vi "QAM Single Carrier.vi"(4 "Symbol Rate":i32=1, 5 "Samples/Symbol":i32, 6 "DataLen":i32, 7 "QAM Comparison":enum16{"MT Modulate", "Homebrew"}(ring), 8 "QAM Complexity":T1(ring)) -> (0 "sampling info":cluster{"Fs":dbl, "#s":dbl}={"Fs"=1000.0, "#s"=1000.0} {"Fs" format="%.2p"}, 1 "Waveform Graph":cluster{"t0":dbl, "dt":dbl, "Y":dbl[]}(graph), 2 "Waveform":waveform(cdb), 3 "Constellation Graph":T2(graph))   [LabVIEW 2018]
uses:
  <vilib>/addons/Modulation/Analog/support/mod_Set Error Source.vi
  <vilib>/Utility/file.llb/Read Delimited Spreadsheet (DBL).vi
  <vilib>/addons/Modulation/Digital/Support/Common/Validators/mod_Generate Filter Coefficients Validate.vi
  <vilib>/addons/Modulation/Digital/General/subVIs/mod_Generate Filter Coefficients.vi
  <vilib>/addons/Modulation/niDMT.lvlib
panel:
  out "size(s)":i32
  out "Array - Numeric":cdb[](array[numeric])
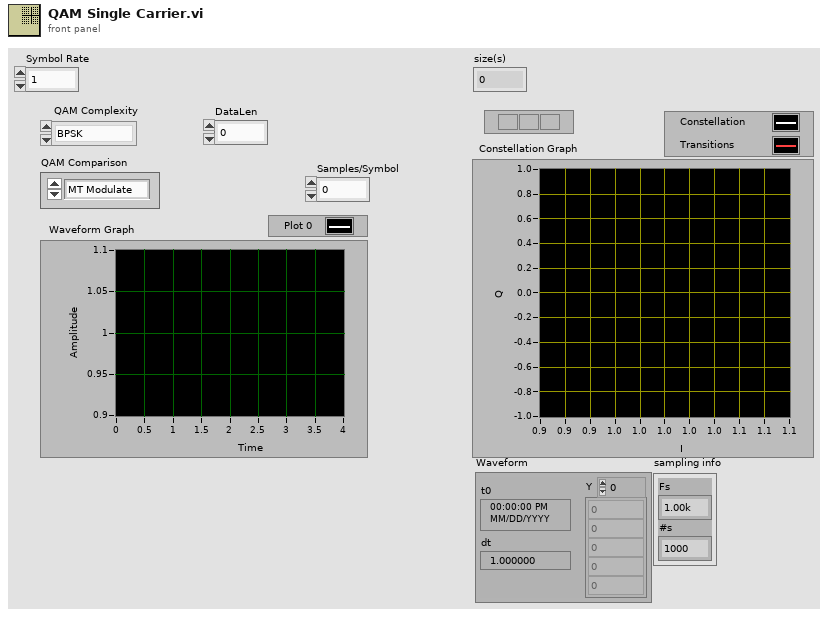
[diagram p1: front panel]
types:
  T1 = enum16{"BPSK", "QPSK", "16-QAM", "64-QAM", "256-QAM"}
  T2 = cluster{"Decimated Array":dbl[], "Decimated Array":dbl[]}[]
  T3 = cluster{"Samples/Symbol":i32, "Array - Numeric":cdb[]}
  T4 = enum16{"FSK", "PSK", "QAM", "MSK", "PAM", "ASK", "CPM"}
  T5 = typedef "niAMT.lvlib/Complex Data Waveform.ctl" = cluster{"t0":dbl, "dt":dbl, "Y":cdb[]}
  T6 = cluster{"constellation":dbl[], "oversampled data":dbl[]}[]
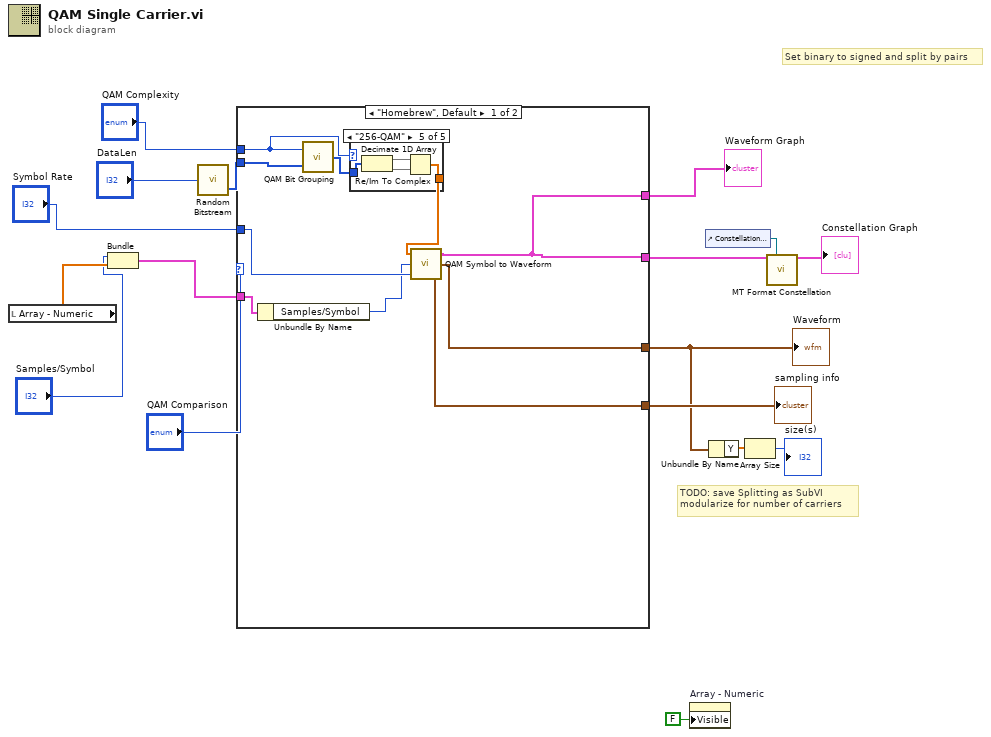
[diagram p0: block diagram]
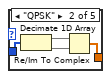
[diagram p3: hidden frame]
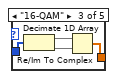
[diagram p4: hidden frame]
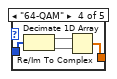
[diagram p5: hidden frame]
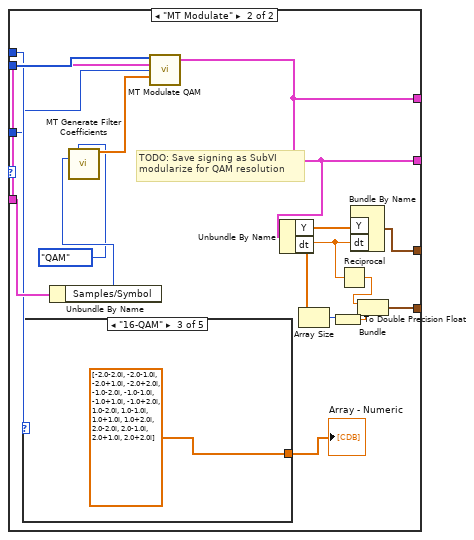
[diagram p6: hidden frame]
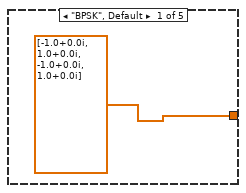
[diagram p7: hidden frame]
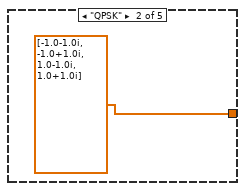
[diagram p8: hidden frame]
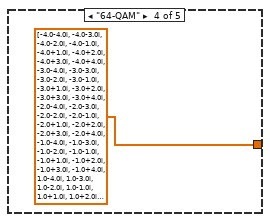
[diagram p9: hidden frame]
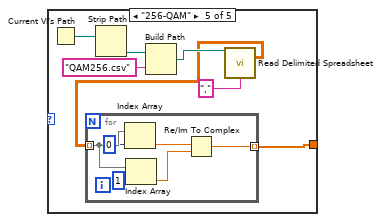
[diagram p10: hidden frame]
diagram:
  # "TODO: save Splitting as SubVI\nmodularize for number of carriers"
  # "Set binary to signed and split by pairs"
  n1 = local read "Array - Numeric"() -> (w8:cdb[])
  n2 = Bundle("Samples/Symbol"="Samples/Symbol", "Array - Numeric"=w8) -> (w7:T3)  [unwired: 1 in]
  n3 = call "Random Bitstream.vi"("DataLen"="DataLen") -> ("Array"=w16:i32[])  [unwired: 1 out]
  n4 = case shown="\"Homebrew\", Default" "QAM Comparison" {
    tunnel: w16 -> [w27 w60]
    tunnel: w7 -> [w20 w58]
    tunnel: [w23 w52] -> w12
    tunnel: [w23 w52] -> w11
    tunnel: "QAM Complexity" -> [w18 w55]
    tunnel: "Symbol Rate" -> [w24 w53]
    tunnel: [w22 w51] -> w3
    tunnel: [w21 w50] -> w5
    frame "Homebrew", Default {
      n5 = Unbundle By Name(w20) -> ("Samples/Symbol"=w19:i32)
      n6 = call "QAM Bit Grouping.vi"("BitStream In"=w27, "QAM Complexity"=w18) -> ("Symbol Out"=w26:i32[])
      n7 = case shown="\"256-QAM\"" w18 {
        tunnel: w26 -> [w28 w32 w36 w40 w44]
        tunnel: [w28 w29 w33 w37 w41] -> w25
        frame "BPSK", Default {
        }
        frame "QPSK" {
          n8 = Decimate 1D Array(w32) -> (w31:i32[], w30:i32[])
          n9 = Re/Im To Complex(1:w30, 2:w31) -> (0:w29:cdb[])
        }
        frame "16-QAM" {
          n10 = Decimate 1D Array(w36) -> (w35:i32[], w34:i32[])
          n11 = Re/Im To Complex(1:w34, 2:w35) -> (0:w33:cdb[])
        }
        frame "64-QAM" {
          n12 = Decimate 1D Array(w40) -> (w39:i32[], w38:i32[])
          n13 = Re/Im To Complex(1:w38, 2:w39) -> (0:w37:cdb[])
        }
        frame "256-QAM" {
          n14 = Decimate 1D Array(w44) -> (w43:i32[], w42:i32[])
          n15 = Re/Im To Complex(1:w42, 2:w43) -> (0:w41:cdb[])
        }
      }
      n16 = call "QAM Symbol to Waveform.vi"("Symbol Rate (Hz)"=w24, "Samples / Symbol"=w19, "Symbol Listing"=w25) -> ("sampling info"=w21:cluster{"Fs":dbl, "#s":dbl}, "Waveform"=w22:waveform(cdb), "output complex waveform"=w23:T5)
    }
    frame "MT Modulate" {
      # "TODO: Save signing as SubVI\nmodularize for QAM resolution"
      n17 = case shown="\"16-QAM\"" w55 {
        tunnel: [cdb[] [-1.0+0.0i, 1.0+0.0i, -1.0+0.0i, 1.0+0.0i] ("symbol map") cdb[] [-1.0-1.0i, -1.0+1.0i, 1.0-1.0i, 1.0+1.0i] ("symbol map") cdb[] [-2.0-2.0i, -2.0-1.0i, -2.0+1.0i, -2.0+2.0i, -1.0-2.0i, -1.0-1.0i, -1.0+1.0i, -1.0+2.0i, 1.0-2.0i, 1.0-1.0i, 1.0+1.0i, 1.0+2.0i, 2.0-2.0i, 2.0-1.0i, 2.0+1.0i, 2.0+2.0i] ("symbol map") cdb[] [-4.0-4.0i, -4.0-3.0i, -4.0-2.0i, -4.0-1.0i, -4.0+1.0i, -4.0+2.0i, -4.0+3.0i, -4.0+4.0i, -3.0-4.0i, -3.0-3.0i, -3.0-2.0i, -3.0-1.0i, -3.0+1.0i, -3.0+2.0i, -3.0+3.0i, -3.0+4.0i, -2.0-4.0i, -2.0-3.0i, -2.0-2.0i, -2.0-1.0i, -2.0+1.0i, -2.0+2.0i, -2.0+3.0i, -2.0+4.0i, -1.0-4.0i, -1.0-3.0i, -1.0-2.0i, -1.0-1.0i, -1.0+1.0i, -1.0+2.0i, -1.0+3.0i, -1.0+4.0i, 1.0-4.0i, 1.0-3.0i, 1.0-2.0i, 1.0-1.0i, 1.0+1.0i, 1.0+2.0i, 1.0+3.0i, 1.0+4.0i, 2.0-4.0i, 2.0-3.0i, 2.0-2.0i, 2.0-1.0i, 2.0+1.0i, 2.0+2.0i, 2.0+3.0i, 2.0+4.0i, 3.0-4.0i, 3.0-3.0i, 3.0-2.0i, 3.0-1.0i, 3.0+1.0i, 3.0+2.0i, 3.0+3.0i, 3.0+4.0i, 4.0-4.0i, 4.0-3.0i, 4.0-2.0i, 4.0-1.0i, 4.0+1.0i, 4.0+2.0i, 4.0+3.0i, 4.0+4.0i] ("symbol map") w66] -> w54
        frame "BPSK", Default {
        }
        frame "QPSK" {
        }
        frame "16-QAM" {
        }
        frame "64-QAM" {
        }
        frame "256-QAM" {
          n18 = Current VI's Path() -> (path=w68:path)
          n19 = Strip Path(path=w68) -> (stripped path=w65:path)  [unwired: 1 out]
          n20 = Build Path(base path=w65, name or relative path="QAM256.csv") -> (appended path=w70:path)
          n21 = call-poly <vilib>:"Read Delimited Spreadsheet.vi"("file path (dialog if empty)"=w70, "delimiter (\\t)"="," ("delimiter (\\t)")) -> ("all rows"=w67:dbl[][])  [unwired: 8 in, 5 out]
          n22 = for {
            tunnel: w67 -> [w77] mode=indexing
            tunnel: [w72] -> w66 mode=indexing
            n23 = Index Array(array=w77, index=0) -> (element=w74:dbl)
            n24 = Index Array(array=w77, index=1) -> (element=w73:dbl)
            n25 = Re/Im To Complex(1:w73, 2:w74) -> (0:w72:cdb)
          }
        }
      }
      "Array - Numeric" <- w54
      n26 = Unbundle By Name(w58) -> ("Samples/Symbol"=w57:i32)
      n27 = call <vilib>:"MT Generate Filter Coefficients.vi"("modulation type"=T4."QAM", "pulse shaping samples per symbol (16)"=w57) -> ("pulse shaping filter coefficients"=w59:dbl[])  [unwired: 11 in, 2 out]
      n28 = call <vilib>:"MT Modulate QAM.vi"("input bit stream"=w60, "QAM system parameters"=w58, "symbol rate (Hz)"=w53, "pulse shaping filter coefficients"=w59) -> ("output complex waveform"=w52:T5)  [unwired: 9 in, 2 out]
      n29 = Unbundle By Name(w52) -> ("Y"=w49:cdb[], "dt"=w47:dbl)
      n30 = Array Size(array=w49) -> (size(s)=w46:i32)
      n31 = To Double Precision Float(number=w46) -> (double precision float=w45:dbl)
      n32 = Reciprocal(x=w47) -> (1/x=w48:dbl)
      n33 = Bundle By Name("Y"=w49, "dt"=w47) -> (w51:waveform(cdb))  [unwired: 1 in]
      n34 = Bundle(w48, w45) -> (w50:cluster{dbl, dbl})  [unwired: 1 in]
    }
  }
  "Waveform Graph" <- w12
  "Waveform" <- w3
  "sampling info" <- w5
  n35 = property on="Array - Numeric" class="Arr (strict)"("Visible"=FALSE) -> ()  [unwired: 2 in, 2 out]
  n36 = control-ref of="Constellation Graph"() -> (w15:refnum<vi>)
  n37 = Unbundle By Name(w3) -> ("Y"=w2:cdb[])
  n38 = Array Size(array=w2) -> (size(s)=→"size(s)":i32)
  n39 = call <vilib>:"MT Format Constellation.vi"("waveform"=w11, "constellation reference"=w15) -> ("constellation graph"=→"Constellation Graph":T6)  [unwired: 3 in, 10 out]
